vi "Check Unicode Response HÜll°.vi"() -> ()   [LabVIEW 2015, in "Integrations.lvlib"]
uses:
  Integrations.lvlib
  <vilib>/Wiresmith Technology/G CLI/CLI Class/CLI.lvclass
panel:
  out "error out":errorcluster
  out "Custom Parameters":string[](array[string])
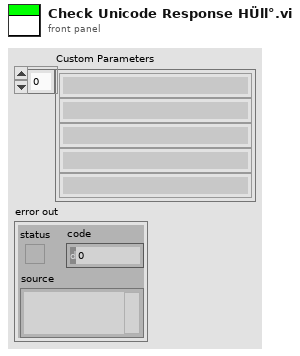
[diagram p1: front panel]
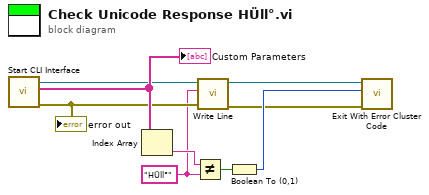
[diagram p0: block diagram]
diagram:
  w1 = "HÜll°"
  n1 = call <vilib>:"Start CLI Interface.vi"() -> ("error out"=w2:errorcluster, "Custom Parameters"=w9:string[], "CLI out"=w3:refnum<class "CLI.lvclass">)  [unwired: 8 in, 1 out]
  "Custom Parameters" <- w9
  "error out" <- w2
  n2 = Index Array(array=w9) -> (element=w8:string)  [unwired: 1 in]
  n3 = Not Equal?(x=w8, y=w1) -> (x != y?=w7:bool)
  n4 = call <vilib>:"Write Line.vi"("error in (no error)"=w2, "Text to Write"=w1, "CLI in"=w3) -> ("error out"=w5:errorcluster, "CLI out"=w4:refnum<class "CLI.lvclass">)  [unwired: 7 in]
  n5 = Boolean To (0,1)(Boolean=w7) -> (0, 1=w6:i16)
  n6 = call <vilib>:"Exit With Error Cluster Code.vi"("error in (no error)"=w5, "No Error Code (0)"=w6, "CLI in"=w4) -> ()  [unwired: 8 in, 1 out]
